vi "Ground Intake Controls.vi"(8 "Stored Game Piece":T1, 9 "Deadband":dbl=0.2 format="%#_13g", 10 "Driver Buttons":bool[](array[boolean]), 11 "Driver Axes":dbl[](array[numeric])) -> (3 "Is Idle?":bool)   [LabVIEW 2020]
uses:
  manipulator/Implementation/Typedefs/game object.ctl
  intake sub/Implementation/intake sub Operations.ctl
  intake sub/Implementation/Typedef/intake typedef.ctl
  <vilib>/Rock Robotics/WPI/Utilities/WPI_GetSetVariantRefNum.vi
  Framework/Robot Global Data.vi
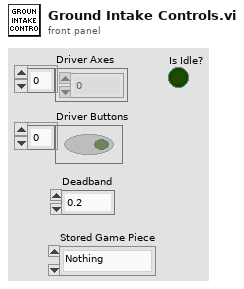
[diagram p1: front panel]
types:
  T1 = typedef "game object.ctl" = enum16{"Nothing", "Cone", "Cube"}
  T2 = typedef "intake typedef.ctl" = enum16{"Intake Cone Sideways", "Intake Cone Upright", "Intake Cube", "Outtake/Score", "Shoot"}
  T3 = typedef "intake sub Operations.ctl" = enum16{"Reserve", "Read Current", "Immediate"}
  T4 = typedef "WPI_JoystickDevRef.ctl" = cluster{"Device":T5}
  T5 = typedef "WPI_JoystickDeviceEnum.ctl" = enum16{"USB 0", "USB 1", "USB 2", "USB 3", "USB 4", "USB 5"}
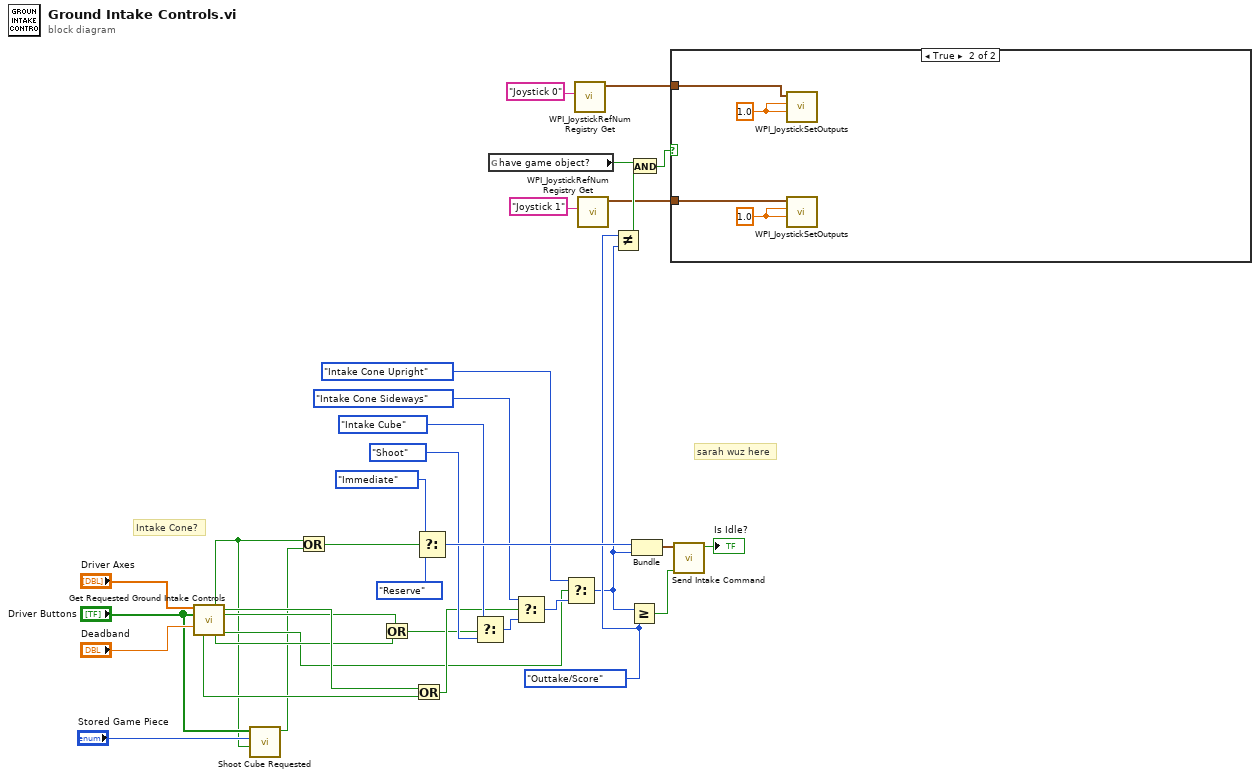
[diagram p0: block diagram]
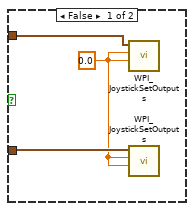
[diagram p2: hidden frame]
diagram:
  w21 = intake_typedef."Outtake/Score" ("y")
  # "sarah wuz here"
  # "Intake Cone?"
  n1 = call "Get Requested Ground Intake Controls.vi"("Driver Axes"="Driver Axes", "Driver Buttons"="Driver Buttons", "Deadband"="Deadband") -> ("Intake Command Requested?"=w10:bool, "Intake Sideways Cone Requested?"=w19:bool, "Intake Cube Requested?"=w14:bool, "Intake Cone Feeder"=w18:bool, "Intake Cube Feeder"=w16:bool, "Intake Upright Cone Requested?"=w15:bool)  [unwired: 6 in, 1 out]
  n2 = call "Shoot Cube Requested.vi"("Other Command Requested?"=w10, "Stored Game Piece"="Stored Game Piece", "Driver Buttons"="Driver Buttons") -> ("Shoot Cube Requested?"=w8:bool)  [unwired: 7 in, 1 out]
  n3 = Or(x=w10, y=w8) -> (x .or. y?=w9:bool)
  n4 = Or(x=w14, y=w16) -> (x .or. y?=w13:bool)
  n5 = Or(x=w19, y=w18) -> (x .or. y?=w17:bool)
  n6 = Select(t=intake_sub_Operations."Immediate" ("Enum"), s=w9, f=intake_sub_Operations."Reserve" ("Enum")) -> (s? t:f=w30:T3)
  n7 = Select(t=intake_typedef."Intake Cube" ("intake modes"), s=w13, f=intake_typedef."Shoot") -> (s? t:f=w33:T2)
  n8 = global read "Robot Global Data.vi" "have game object?"() -> (w1:bool)
  n9 = Select(t=intake_typedef."Intake Cone Sideways" ("intake modes"), s=w17, f=w33) -> (s? t:f=w23:T2)
  n10 = Select(t=intake_typedef."Intake Cone Upright", s=w15, f=w23) -> (s? t:f=w20:T2)
  n11 = call <vilib>:"WPI_JoystickRefNum Registry Get.vi"("refnum name"="Joystick 0") -> ("JoystickDevRef"=w5:T4)  [unwired: 1 in, 9 out]
  n12 = call <vilib>:"WPI_JoystickRefNum Registry Get.vi"("refnum name"="Joystick 1") -> ("JoystickDevRef"=w3:T4)  [unwired: 1 in, 9 out]
  n13 = Not Equal?(x=w21, y=w20) -> (x != y?=w6:bool)
  n14 = Greater Or Equal?(x=w20, y=w21) -> (x >= y?=w24:bool)
  n15 = And(x=w1, y=w6) -> (x .and. y?=w7:bool)
  n16 = Bundle("Enum"=w30, "f"=w20) -> (w27:cluster{"Enum":T3, "f":T2})  [unwired: 1 in]
  n17 = case shown="True" w7 {
    tunnel: w3 -> [w38 w42]
    tunnel: w5 -> [w36 w41]
    frame False {
      w37 = sgl 0.0 ("Left Rumble")
      n18 = call <vilib>:"WPI_JoystickSetOutputs.vi"("Right Rumble"=w37, "Left Rumble"=w37, "JoystickDevRef"=w36) -> ()  [unwired: 7 in, 2 out]
      n19 = call <vilib>:"WPI_JoystickSetOutputs.vi"("Right Rumble"=w37, "Left Rumble"=w37, "JoystickDevRef"=w38) -> ()  [unwired: 7 in, 2 out]
    }
    frame True {
      w39 = sgl 1.0 ("Left Rumble")
      w40 = sgl 1.0 ("Left Rumble")
      n20 = call <vilib>:"WPI_JoystickSetOutputs.vi"("Right Rumble"=w40, "Left Rumble"=w40, "JoystickDevRef"=w41) -> ()  [unwired: 7 in, 2 out]
      n21 = call <vilib>:"WPI_JoystickSetOutputs.vi"("Right Rumble"=w39, "Left Rumble"=w39, "JoystickDevRef"=w42) -> ()  [unwired: 7 in, 2 out]
    }
  }
  n22 = call "Send Intake Command.vi"("Wait for Manipulator"=w24, "Intake Command"=w27) -> ("Is Idle?"=→"Is Idle?":bool)  [unwired: 9 in]
